vi "SetArmSpikeMotors.vi"(8 "Direction For Right":T1, 9 "Direction For Left":T1, 11 "Name":string) -> (0 "error out":errorcluster)   [LabVIEW 2013]
uses:
  <vilib>/Rock Robotics/WPI/Relay/WPI_RelayValue.ctl
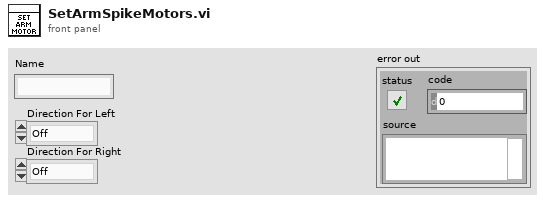
[diagram p1: front panel]
types:
  T1 = typedef "WPI_RelayValue.ctl" = enum16{"Off", "On", "Forward", "Reverse"}
  T2 = typedef "WPI_RelayDevRef.ctl" = cluster{"DevStatus":errorcluster, "Relay Channel":T3, "Digital Module":T4, "Relay Direction":T5}
  T3 = typedef "FPGA_DIORelayChannel.ctl" = enum8{"Relay 1", "Relay 2", "Relay 3", "Relay 4", "Relay 5", "Relay 6", "Relay 7", "Relay 8", "Invalid"}
  T4 = typedef "FPGA_TypedefDigitalModule.ctl" = enum16{"Digital Module 1", "Digital Module 2"}
  T5 = typedef "WPI_RelayDirection.ctl" = enum16{"Both directions", "Forward only", "Reverse only"}
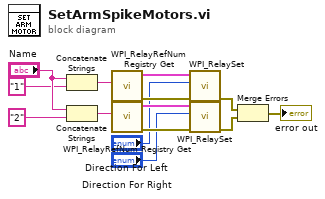
[diagram p0: block diagram]
diagram:
  n1 = Concatenate Strings("Name", "1") -> (w14:string)
  n2 = Concatenate Strings("Name", "2" ("string")) -> (w13:string)
  n3 = call <vilib>:"WPI_RelayRefNum Registry Get.vi"("refnum name"=w14) -> ("error out"=w9:errorcluster, "RelayDevRef"=w8:T2)  [unwired: 9 in]
  n4 = call <vilib>:"WPI_RelayRefNum Registry Get.vi"("refnum name"=w13) -> ("error out"=w6:errorcluster, "RelayDevRef"=w7:T2)  [unwired: 9 in]
  n5 = call <vilib>:"WPI_RelaySet.vi"("error in (no error)"=w9, "RelayValue"="Direction For Left", "RelayDevRef"=w8) -> ("error out"=w5:errorcluster)  [unwired: 7 in, 1 out]
  n6 = call <vilib>:"WPI_RelaySet.vi"("error in (no error)"=w6, "RelayValue"="Direction For Right", "RelayDevRef"=w7) -> ("error out"=w4:errorcluster)  [unwired: 7 in, 1 out]
  n7 = Merge Errors(w5, w4) -> (→"error out":errorcluster)
